vi "NI-DAQ RUS Lockin.vi"(6 "Init?":bool, 8 "error in (no error)":errorcluster, 11 "RUS settings":T1={"NI-DAQ lockin settings"={"Samples per sine wave"=0, "Sine waves per freq step"=0, "Output Representation"=enum."Real/Imaginary", "Low-pass filter"=enum."Butterworth", "Ranges and couplings "=[]}, "Fast swep settings"={"Update rate (Hz)"=250.0, "Start F, Hz"=200000.0, "Stop F"=1700000.0, "Number of points"=30000, "Amplitude"=2.1, "Init&amplitude"=TRUE, "IF"=1000.0, "Time constant"=0.1}, "Pre-sweep delay, s"=0.0, "Lockin mode"=enum."NI-DAQ", "SR Lockin"="GPIB0::10::INSTR", "DAQmx Device"="Dev3", "Clock Multiplier"=64, "Fast Sweep Data Out"={"DO clock task"="", "DO task"="", "Update clock task"="", "DAQ lockin task"="", "Pre-sweep counter task"=""}, "Lockin Range, V"=0.0, "F Array"=[], "Freq. update clock terminal"="", "DO Clock Rate (Hz)"=5000000.0, "ADC clock terminal"="/PFI4", "Pre-sweep counter terminal"="/PFI4", "Samples per read"=10, "DO clock terminal"="", "Pre-sweep points"=0, "F points per write"=0, "Total sweep time, s"=1000.0, "Initial SYNTH phase"=0.0, "Record IF"=FALSE, "Save data settings"={"Save data"=TRUE, "Data Root Path"=path "", "File Prefix"="", "File Format"=enum."ASCII", "Save column names"=TRUE, "File Comments"="<Description of the current file>", "User/Prj"="<User Name/Project Description>"}, "Data file path"=path "", "New data user event"=refnum, "Stop user event"=refnum, "Number of channels"=1, "Auto-phase"=FALSE} {"Lockin Range, V" format="%#_6e"; "Fast swep settings"."IF" format="%#_6p"; "Fast swep settings"."Amplitude" min=0.0 max=2.5; "Fast swep settings"."Number of points" format="%.0p"; "Fast swep settings"."Stop F" format="%#_6p"; "Fast swep settings"."Start F, Hz" format="%#_6p"; "Fast swep settings"."Update rate (Hz)" format="%0.2f"; "NI-DAQ lockin settings"."Ranges and couplings"."Coupling" items=["default"=-1, "RSE"=10083, "NRSE"=10078, "Differential"=10106, "Pseudodifferential"=12529]}) -> (0 "error out":errorcluster, 1 "AvailSampPerChan":u32, 3 "RUS settings out":T1={"NI-DAQ lockin settings"={"Samples per sine wave"=0, "Sine waves per freq step"=0, "Output Representation"=enum."Real/Imaginary", "Low-pass filter"=enum."Butterworth", "Ranges and couplings "=[]}, "Fast swep settings"={"Update rate (Hz)"=250.0, "Start F, Hz"=200000.0, "Stop F"=1700000.0, "Number of points"=30000, "Amplitude"=2.1, "Init&amplitude"=TRUE, "IF"=1000.0, "Time constant"=0.1}, "Pre-sweep delay, s"=0.0, "Lockin mode"=enum."NI-DAQ", "SR Lockin"="GPIB0::10::INSTR", "DAQmx Device"="Dev3", "Clock Multiplier"=64, "Fast Sweep Data Out"={"DO clock task"="", "DO task"="", "Update clock task"="", "DAQ lockin task"="", "Pre-sweep counter task"=""}, "Lockin Range, V"=0.0, "F Array"=[], "Freq. update clock terminal"="", "DO Clock Rate (Hz)"=5000000.0, "ADC clock terminal"="/PFI4", "Pre-sweep counter terminal"="/PFI4", "Samples per read"=10, "DO clock terminal"="", "Pre-sweep points"=0, "F points per write"=0, "Total sweep time, s"=1000.0, "Initial SYNTH phase"=0.0, "Record IF"=FALSE, "Save data settings"={"Save data"=TRUE, "Data Root Path"=path "", "File Prefix"="", "File Format"=enum."ASCII", "Save column names"=TRUE, "File Comments"="<Description of the current file>", "User/Prj"="<User Name/Project Description>"}, "Data file path"=path "", "New data user event"=refnum, "Stop user event"=refnum, "Number of channels"=1, "Auto-phase"=FALSE} {"Lockin Range, V" format="%#_6e"; "Fast swep settings"."IF" format="%#_6p"; "Fast swep settings"."Amplitude" min=0.0 max=2.5; "Fast swep settings"."Number of points" format="%.0p"; "Fast swep settings"."Stop F" format="%#_6p"; "Fast swep settings"."Start F, Hz" format="%#_6p"; "Fast swep settings"."Update rate (Hz)" format="%0.2f"; "NI-DAQ lockin settings"."Ranges and couplings"."Coupling" items=["default"=-1, "RSE"=10083, "NRSE"=10078, "Differential"=10106, "Pseudodifferential"=12529]}, 5 "Lockin out":dbl[][](array[numeric]))   [LabVIEW 2015]
uses:
  Controls/RUS settings.ctl
  Controls/RUS NI-DAQ Lockin Settings.ctl
  Controls/Sweep settings.ctl
  NHMFL_Core/Libraries/File/Controls/Save data settings.ctl
  NHMFL_Core/Libraries/File/Controls/File formats.ctl
  Multi-Channel Lockin/Controls/Lockin Settings.ctl
  Multi-Channel Lockin/Controls/Harmonics per channel.ctl
  <vilib>/Analysis/2dsp.llb/Decimate (single shot, DBL).vi
  <vilib>/Analysis/NI_AALPro.lvlib
  <resource>/objmgr/daqmx.rc
panel:
  out "size(s)":i32[](array[numeric])
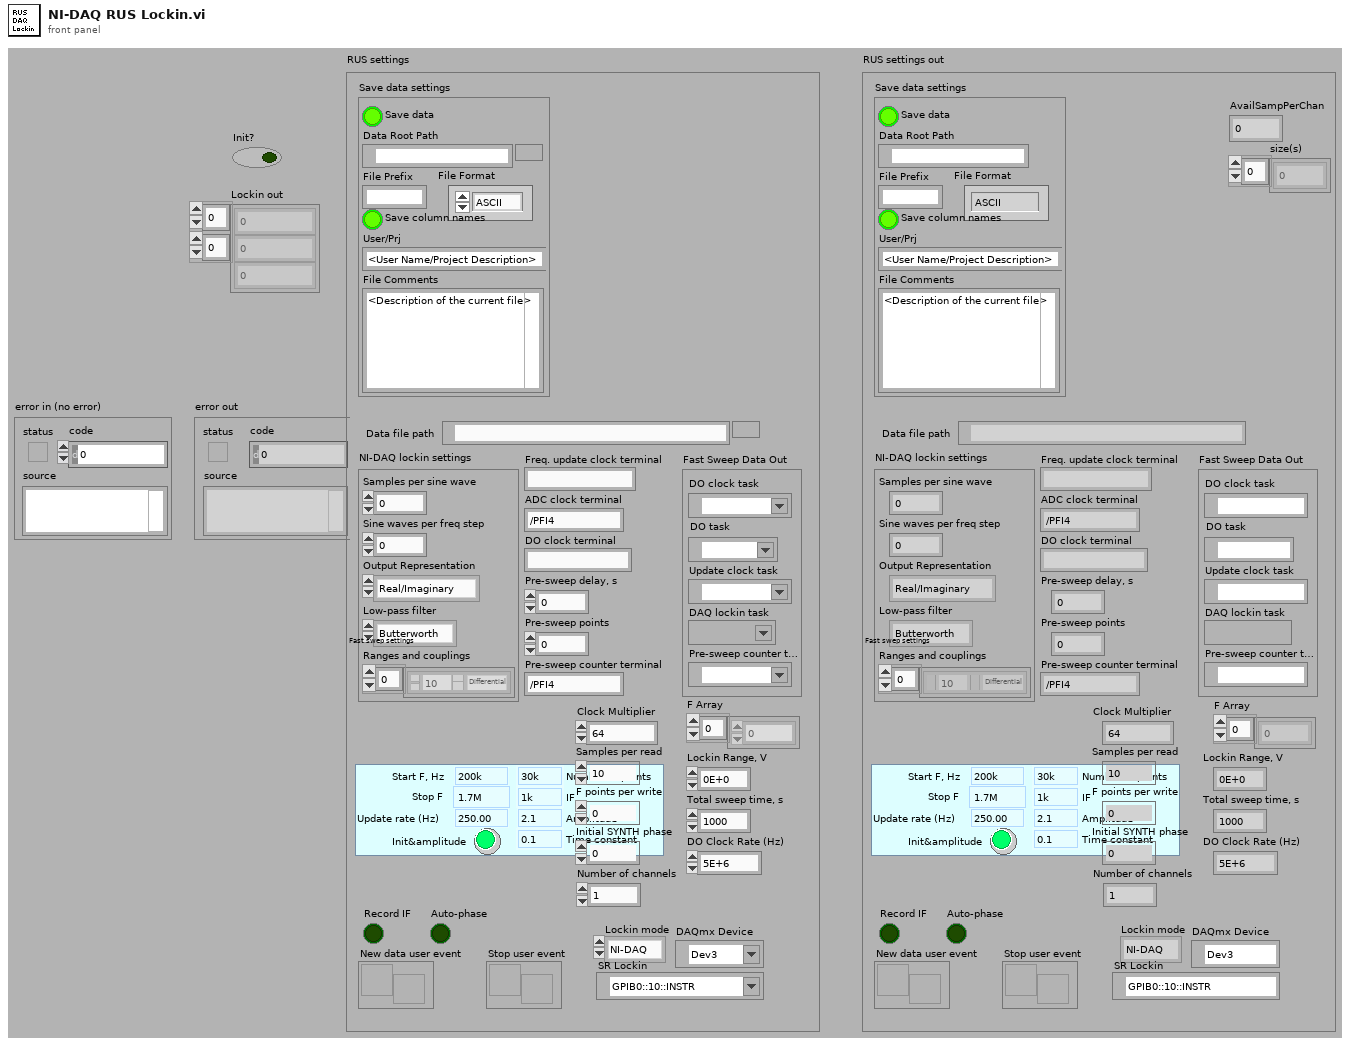
[diagram p1: front panel]
types:
  T1 = typedef "RUS settings.ctl" = cluster{"NI-DAQ lockin settings":T2, "Fast swep settings":T3, "Pre-sweep delay, s":dbl, "Lockin mode":enum16{"SRS", "NI-DAQ"}, "SR Lockin":refnum<visa-resource-name>, "DAQmx Device":tag, "Clock Multiplier":i32, "Fast Sweep Data Out":cluster{"DO clock task":refnum<k21>, "DO task":refnum<k21>, "Update clock task":refnum<k21>, "DAQ lockin task":refnum<k21>, "Pre-sweep counter task":refnum<k21>}, "Lockin Range, V":sgl, "F Array":dbl[], "Freq. update clock terminal":string, "DO Clock Rate (Hz)":dbl, "ADC clock terminal":string, "Pre-sweep counter terminal":string, "Samples per read":i32, "DO clock terminal":string, "Pre-sweep points":i32, "F points per write":i32, "Total sweep time, s":dbl, "Initial SYNTH phase":dbl, "Record IF":bool, "Save data settings":T4, "Data file path":path, "New data user event":refnum<user-event>, "Stop user event":refnum<user-event>, "Number of channels":i32, "Auto-phase":bool}
  T2 = typedef "RUS NI-DAQ Lockin Settings.ctl" = cluster{"Samples per sine wave":i32, "Sine waves per freq step":i32, "Output Representation":enum16{"Real/Imaginary", "Polar"}, "Low-pass filter":enum16{"No filtering", "Butterworth", "Bessel"}, "Ranges and couplings ":cluster{"Range":dbl, "Coupling":i32}[]}
  T3 = typedef "Sweep settings.ctl" = cluster{"Update rate (Hz)":dbl, "Start F, Hz":dbl, "Stop F":dbl, "Number of points":i32, "Amplitude":dbl, "Init&amplitude":bool, "IF":dbl, "Time constant":dbl}
  T4 = typedef "Save data settings.ctl" = cluster{"Save data":bool, "Data Root Path":path, "File Prefix":string, "File Format":T5, "Save column names":bool, "File Comments":string, "User/Prj":string}
  T5 = typedef "File formats.ctl" = enum16{"TDMS", "ASCII", "BINARY"}
  T6 = typedef "Lockin Settings.ctl" = cluster{"Sine Frequency, Hz":dbl, "Time constant, s":dbl, "Low-pass filter":enum16{"No filtering", "Butterworth", "Bessel"}, "Output representation":enum16{"Real/Imaginary", "Polar"}, "Phases, deg":dbl[], "Low-pass filter Order":i32, "Decimating factor":i32, "Samples to Read":i32, "Post-filter decimation":i32, "Blocks to average":i32, "Trig delay, points":i32, "Harmonics per channel":T7, "Amplitude scale":enum16{"Amplitude", "RMS", "Peak-to-Peak"}}
  T7 = typedef "Harmonics per channel.ctl" = cluster{"Harmonics":i32[]}[]
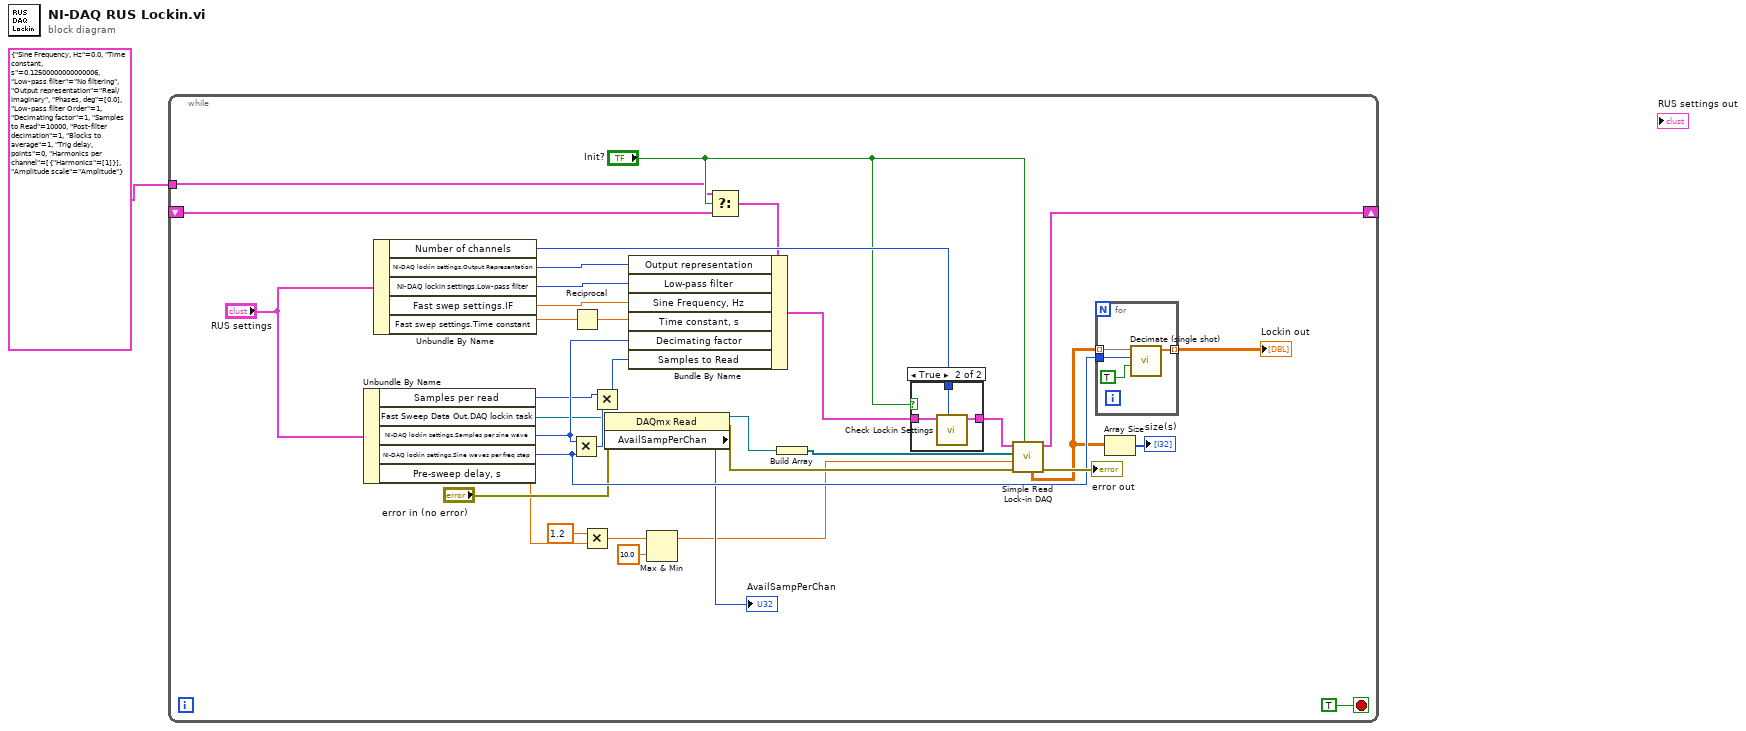
[diagram p0: block diagram]
diagram:
  n1 = while {
    tunnel: T6 {"Sine Frequency, Hz"=0.0, "Time constant, s"=0.12500000000000006, "Low-pass filter"=enum."No filtering", "Output representation"=enum."Real/Imaginary", "Phases, deg"=[0.0], "Low-pass filter Order"=1, "Decimating factor"=1, "Samples to Read"=10000, "Post-filter decimation"=1, "Blocks to average"=1, "Trig delay, points"=0, "Harmonics per channel"=[{"Harmonics"=[1]}], "Amplitude scale"=enum."Amplitude"} ("Lock-in settings") -> [w4]
    shift-right: [w6] -> _
    shift-left: _ -> [w3]
    stop <- TRUE stop-if-true
    n2 = Unbundle By Name("RUS settings") -> ("Samples per read"=w30:i32, "Fast Sweep Data Out.DAQ lockin task"=w28:refnum<k21>, "NI-DAQ lockin settings.Samples per sine wave"=w32:i32, "NI-DAQ lockin settings.Sine waves per freq step"=w29:i32, "Pre-sweep delay, s"=w20:dbl)
    n3 = Unbundle By Name("RUS settings") -> ("Number of channels"=w8:i32, "NI-DAQ lockin settings.Output Representation"=w22:enum16{"Real/Imaginary", "Polar"}, "NI-DAQ lockin settings.Low-pass filter"=w23:enum16{"No filtering", "Butterworth", "Bessel"}, "Fast swep settings.IF"=w10:dbl, "Fast swep settings.Time constant"=w36:dbl)
    n4 = Multiply(x=w32, y=w29) -> (x*y=w33:i32)
    n5 = Reciprocal(x=w36) -> (1/x=w9:dbl)
    n6 = Multiply(x=1.2, y=w20) -> (x*y=w19:dbl)
    n7 = Multiply(x=w30, y=w33) -> (x*y=w31:i32)
    n8 = property class="DAQmx Read"(reference=w28, error in="error in (no error)") -> (reference out=w27:refnum<k21>, error out=w25:errorcluster, "AvailSampPerChan"=→"AvailSampPerChan":u32)
    n9 = Max & Min(x=w19, y=10.0) -> (max(x,y)=w17:dbl)  [unwired: 1 out]
    n10 = Select(t=w4, s="Init?", f=w3) -> (s? t:f=w2:T6)
    n11 = Bundle By Name(cluster=w2, "Output representation"=w22, "Low-pass filter"=w23, "Sine Frequency, Hz"=w10, "Time constant, s"=w9, "Decimating factor"=w32, "Samples to Read"=w31) -> (w12:T6)
    n12 = Build Array(w27) -> (w15:refnum<k21>[])
    n13 = case shown="True" "Init?" {
      tunnel: w12 -> [w37 w40]
      tunnel: [w37 w39] -> w11
      tunnel: w8 -> [_ w38]
      frame False {
      }
      frame True {
        n14 = call "Check Lockin Settings.vi"("Number of channels"=w38, "Lock-in settings"=w40) -> ("Lock-in settings out"=w39:T6)  [unwired: 8 in, 1 out]
      }
    }
    n15 = call "Simple Read  Lock-in DAQ.vi"("Initialize?"="Init?", "error in (no error)"=w25, "DAQ timeout, s"=w17, "DAQ Task Array"=w15, "Lock-in settings"=w11) -> ("error out"=→"error out":errorcluster, "Lock-in settings out"=w6:T6, "signal(s) out"=w14:dbl[][])  [unwired: 4 out]
    n16 = for {
      tunnel: w14 -> [w44] mode=indexing
      tunnel: [w43] -> w13 mode=indexing
      tunnel: w29 -> [w42]
      n17 = call-poly <vilib>:"Decimate (single shot).vi"("averaging"=TRUE, "decimating factor"=w42, "X"=w44) -> ("Decimated Array"=w43:dbl[])  [unwired: 7 in, 1 out]
    }
    "Lockin out" <- w13
    n18 = Array Size(array=w14) -> (size(s)=→"size(s)":i32[])
  }
